vi "啮合 扭矩变化峰值.vi"(10 "扭矩反转":dbl[](array[numeric]), 11 "扭矩正转":dbl[](array[numeric])) -> (2 "反转扭矩变化峰值":dbl, 3 "正转扭矩变化峰值":dbl)   [LabVIEW 2015, in "Logging.lvlib"]
uses:
  Logging.lvlib
  <vilib>/Analysis/NI_AAL_SigProc.lvlib
  <vilib>/Analysis/NI_AALBase.lvlib
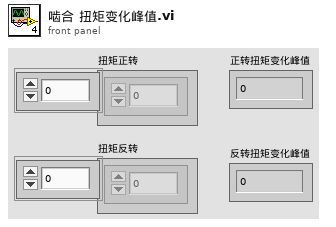
[diagram p1: front panel]
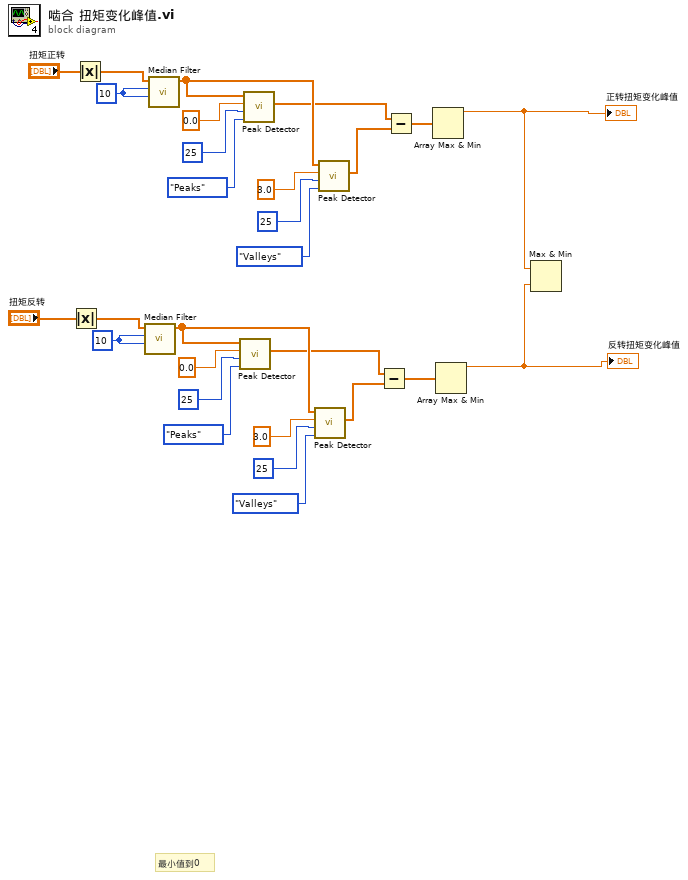
[diagram p0: block diagram]
diagram:
  w17 = 10 ("left rank")
  w28 = 10 ("left rank")
  # "最小值到0"
  n1 = Absolute Value(x="扭矩反转") -> (abs(x)=w9:dbl[])
  n2 = Absolute Value(x="扭矩正转") -> (abs(x)=w20:dbl[])
  n3 = call <vilib>:"Median Filter.vi"("right rank"=w17, "left rank"=w17, "X"=w9) -> ("Filtered X"=w8:dbl[])  [unwired: 7 in, 1 out]
  n4 = call <vilib>:"Median Filter.vi"("right rank"=w28, "left rank"=w28, "X"=w20) -> ("Filtered X"=w19:dbl[])  [unwired: 7 in, 1 out]
  n5 = call <vilib>:"Peak Detector.vi"("peaks/valleys"=enum32{"Peaks", "Valleys"}."Peaks", "width"=25, "threshold"=0.0, "X"=w8) -> ("Amplitudes"=w4:dbl[])  [unwired: 3 in, 4 out]
  n6 = call <vilib>:"Peak Detector.vi"("peaks/valleys"=enum32{"Peaks", "Valleys"}."Peaks", "width"=25, "threshold"=0.0, "X"=w19) -> ("Amplitudes"=w6:dbl[])  [unwired: 3 in, 4 out]
  n7 = call <vilib>:"Peak Detector.vi"("peaks/valleys"=enum32{"Peaks", "Valleys"}."Valleys", "width"=25, "threshold"=3.0, "X"=w8) -> ("Amplitudes"=w3:dbl[])  [unwired: 3 in, 4 out]
  n8 = call <vilib>:"Peak Detector.vi"("peaks/valleys"=enum32{"Peaks", "Valleys"}."Valleys", "width"=25, "threshold"=3.0, "X"=w19) -> ("Amplitudes"=w5:dbl[])  [unwired: 3 in, 4 out]
  n9 = Subtract(x=w4, y=w3) -> (x-y=w7:dbl[])
  n10 = Subtract(x=w6, y=w5) -> (x-y=w18:dbl[])
  n11 = Array Max & Min(array=w18) -> (max value=w2:dbl)  [unwired: 3 out]
  "正转扭矩变化峰值" <- w2
  n12 = Array Max & Min(array=w7) -> (max value=w1:dbl)  [unwired: 3 out]
  "反转扭矩变化峰值" <- w1
  n13 = Max & Min(x=w2, y=w1) -> ()  [unwired: 2 out]
